vi "EuniceF_Project7_Labview - Copy.vi"() -> ()   [LabVIEW 2025]
panel:
  out "Vtc,mV":u8(slide) scale=0.0..100.0
  out "TemperatureChart":dbl(graph)
  out "Vref,mV":dbl(slide) scale=0.0..100.0
  out "Vdiff,mV":dbl(slide) scale=0.0..100.0
  in  "STOP":bool
  out "Thermometer":dbl(slide) scale=0.0..100.0
  out "Vscc,V":dbl(slide) scale=-10.0..10.0
  out "AtoD":i16
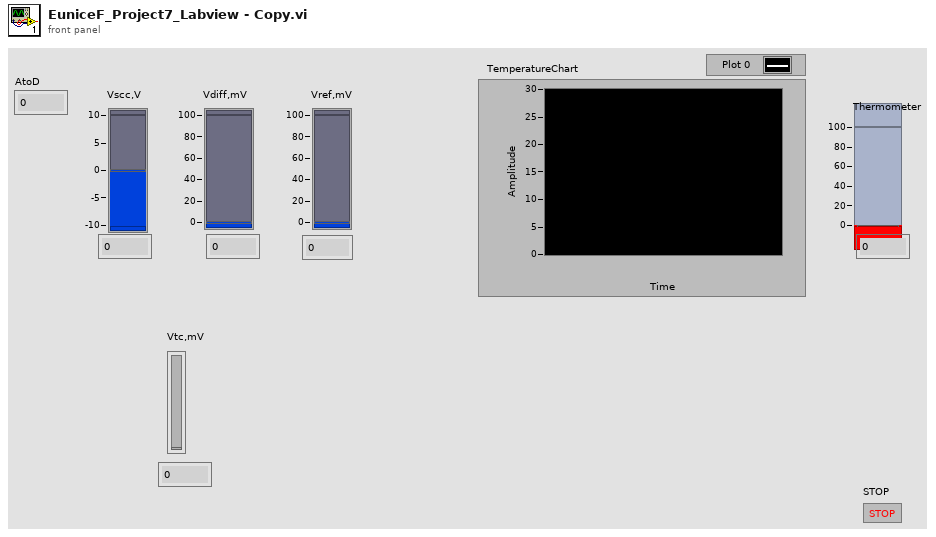
[diagram p1: front panel]
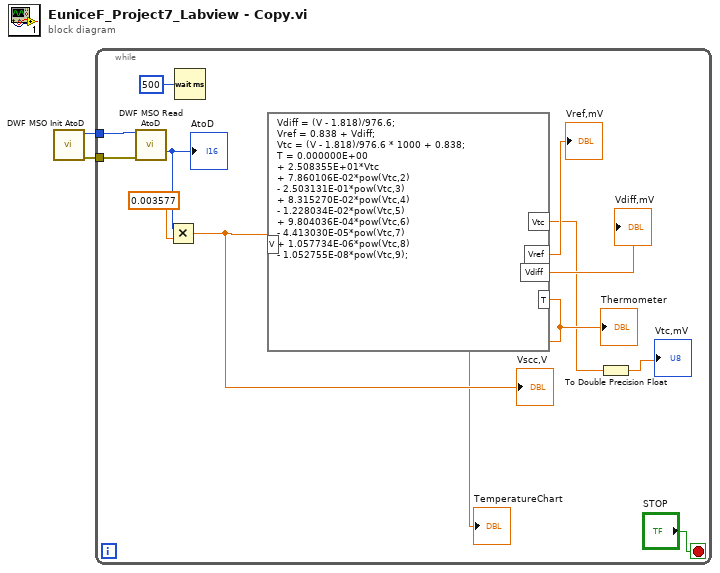
[diagram p0: block diagram]
diagram:
  n1 = call "DWF MSO Init AtoD.vi"() -> ("Error Out"=w1:errorcluster, "Instrument Handle Out"=w2:i32)  [unwired: 10 in]
  n2 = while {
    tunnel: w2 -> [w14]
    tunnel: w1 -> [w13]
    stop <- "STOP" stop-if-true
    n3 = call "DWF MSO Read AtoD.vi"("Instrument Handle In AtoD"=w14, "Error In"=w13) -> ("AtoD"=w12:i16)  [unwired: 12 in, 1 out]
    "AtoD" <- w12
    n4 = Multiply(x=w12, y=0.003577) -> (x*y=w10:dbl)
    "Vscc,V" <- w10
    n5 = Wait (ms)(milliseconds to wait=u32 500) -> ()  [unwired: 1 out]
    n6 = formula code="Vdiff = (V - 1.818)/976.6;\nVref = 0.838 + Vdiff;\nVtc = (V - 1.818)/976.6 * 1000 + 0.838;\nT = 0.000000E+00\n+ 2.508355E+01*Vtc\n+ 7.860106E-02*pow(Vtc,2)\n- 2.503131E-01*pow(Vtc,3)\n+ 8.315270E-02*pow(Vtc,4)\n- 1.228034E-02*pow(Vtc,5)\n+ 9.804036E-04*pow(Vtc,6)\n- 4.413030E-05*pow(Vtc,7)\n+ 1.057734E-06*pow(Vtc,8)\n- 1.052755E-08*pow(Vtc,9);"("V"=w10) -> ("T"=→"Thermometer" →"TemperatureChart":dbl, "Vdiff"=→"Vdiff,mV":dbl, "Vref"=→"Vref,mV":dbl, "Vtc"=w3:dbl)
    n7 = To Double Precision Float(number=w3) -> (double precision float=→"Vtc,mV":dbl)
  }
